vi "CalcSides.vi"(7 "Garden":u8[][](array[numeric]), 11 "Cluster":T1) -> (3 "Numeric":u64)   [LabVIEW 2023, in "2024_12.lvclass"]
uses:
  2024_12.lvclass
panel:
  out "Array":bool[][](array[boolean])
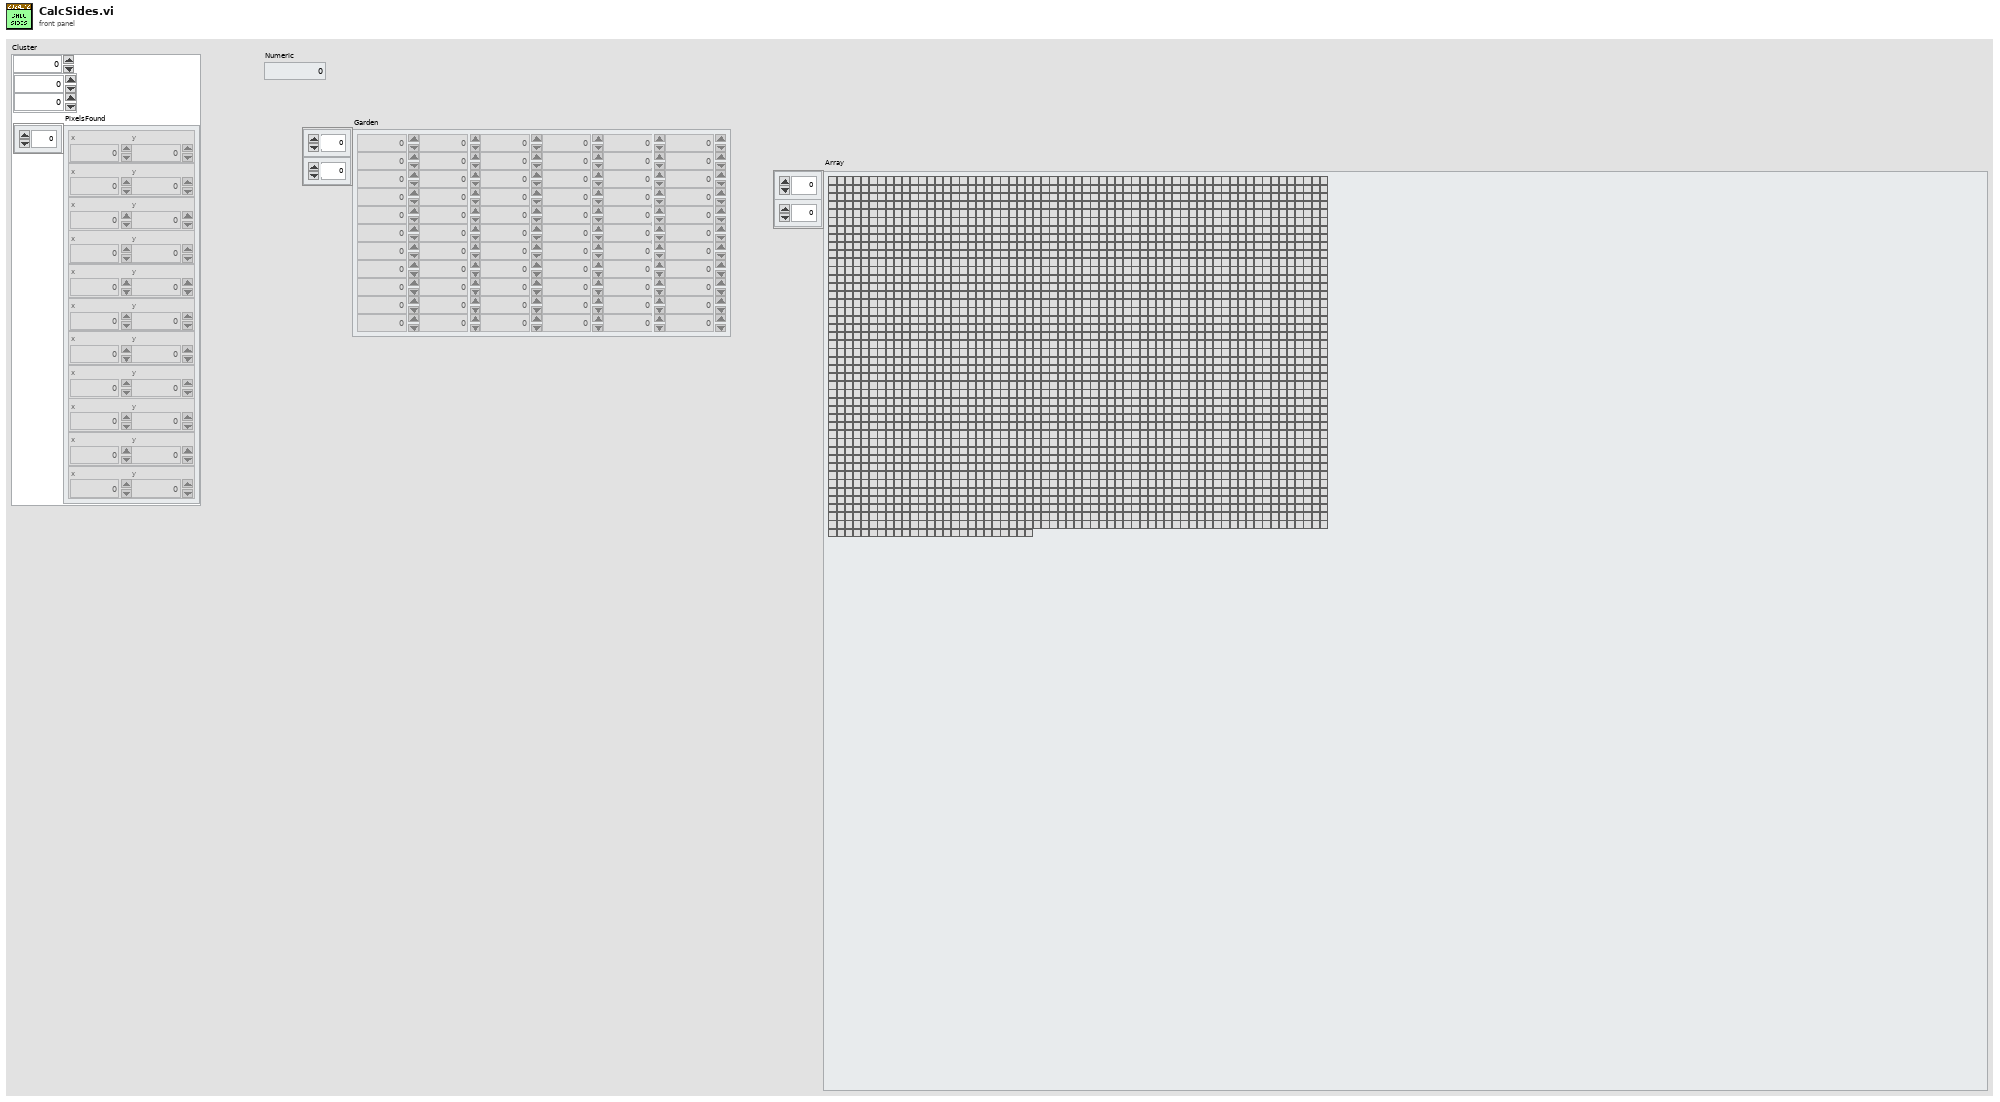
[diagram p1: front panel]
types:
  T1 = cluster{"Numeric":u8, "Cluster":cluster{"Numeric":i32, "Numeric":i32}, "PixelsFound":cluster{"x":i32, "y":i32}[]}
  T2 = cluster{"Start Position":cluster{"x":i32, "y":i32}, enum16{"Left", "Up", "Right", "Down"}, i32}
  T3 = cluster{"Start Position":cluster{"x":i32, "y":i32}, enum16{"Left", "Up", "Right", "Down"}, i32}[]
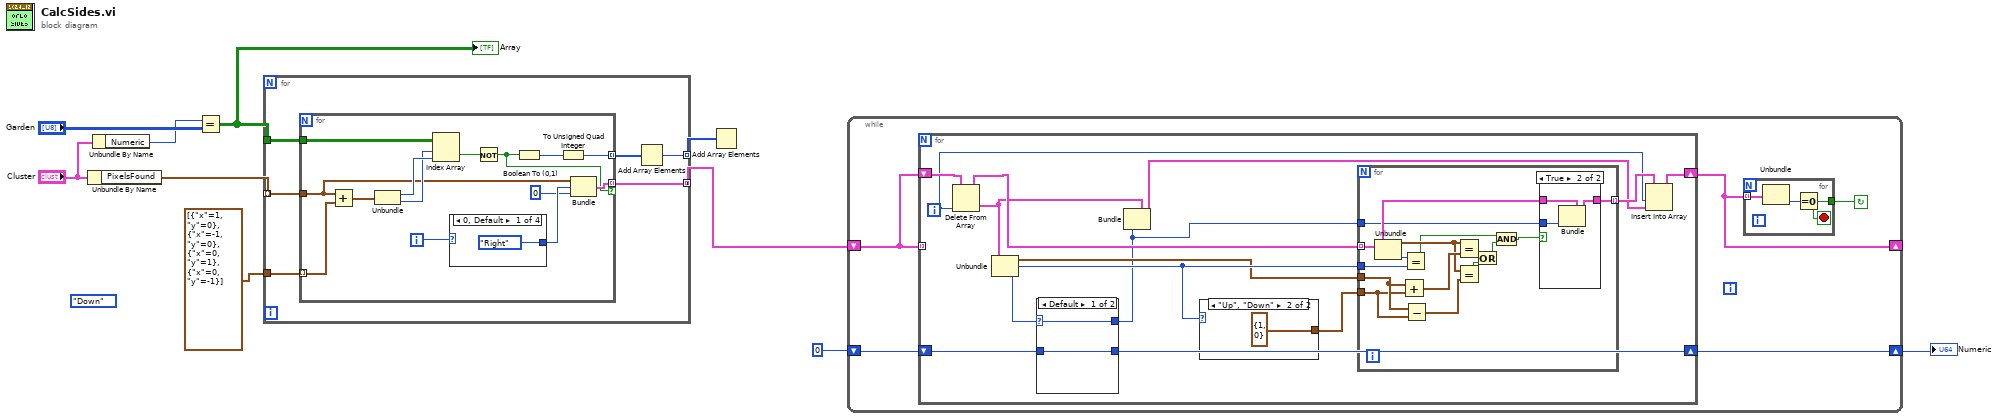
[diagram p0: block diagram]
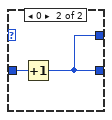
[diagram p2: hidden frame]
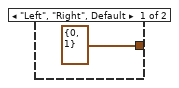
[diagram p4: hidden frame]
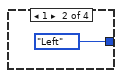
[diagram p5: hidden frame]
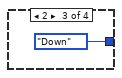
[diagram p6: hidden frame]
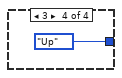
[diagram p7: hidden frame]
diagram:
  (unwired) enum16{"Left", "Up", "Right", "Down"}."Down"
  n1 = Unbundle By Name("Cluster") -> ("PixelsFound"=w10:cluster{"x":i32, "y":i32}[])
  n2 = Unbundle By Name("Cluster") -> ("Numeric"=w7:u8)
  n3 = Equal?(x=w7, y="Garden") -> (x = y?=w4:bool[][])
  "Array" <- w4
  n4 = for {
    tunnel: w10 -> [w15] mode=indexing
    tunnel: w4 -> [w16]
    tunnel: cluster{"x":i32, "y":i32}[] [{"x"=1, "y"=0}, {"x"=-1, "y"=0}, {"x"=0, "y"=1}, {"x"=0, "y"=-1}] ("PixelsFound") -> [w14]
    tunnel: [w12] -> w5 mode=indexing
    tunnel: [w11] -> w3 mode=concatenating
    n5 = for {
      tunnel: w16 -> [w30]
      tunnel: w15 -> [w21]
      tunnel: w14 -> [w29] mode=indexing
      tunnel: [w23] -> w13 mode=indexing
      tunnel: [w19] -> w11 mode=indexing if=w18
      i -> [w22]
      n6 = Add(x=w21, y=w29) -> (x+y=w28:cluster{"x":i32, "y":i32})
      n7 = Unbundle(w28) -> ("x"=w27:i32, "y"=w26:i32)
      n8 = Index Array(array=w30, index (row)=w26, index (col)=w27) -> (element=w25:bool)
      n9 = case shown="0, Default" w22 {
        tunnel: [enum16{"Left", "Up", "Right", "Down"}."Right" enum16{"Left", "Up", "Right", "Down"}."Left" enum16{"Left", "Up", "Right", "Down"}."Down" enum16{"Left", "Up", "Right", "Down"}."Up"] -> w20
        frame 0, Default {
        }
        frame 1 {
        }
        frame 2 {
        }
        frame 3 {
        }
      }
      n10 = Not(x=w25) -> (.not. x?=w18:bool)
      n11 = Boolean To (0,1)(Boolean=w18) -> (0, 1=w24:i16)
      n12 = To Unsigned Quad Integer(1:w24) -> (0:w23:u64)
      n13 = Bundle("Start Position"=w21, w20, 0) -> (w19:T2)  [unwired: 1 in]
    }
    n14 = Add Array Elements(numeric array=w13) -> (sum=w12:u64)
  }
  n15 = Add Array Elements(numeric array=w5) -> ()  [unwired: 1 out]
  n16 = while {
    shift-right: [w36] -> _
    shift-left: w3 -> [w38]
    shift-right: [w37] -> w1
    shift-left: 0 ("index") -> [w39]
    stop <- w35 continue-if-true
    n17 = for {
      tunnel: w38 -> [_] mode=indexing
      shift-right: [w48] -> w36
      shift-left: w38 -> [w50]
      shift-right: [w43] -> w37
      shift-left: w39 -> [w51]
      i -> [w47]
      n18 = Delete From Array(array=w50, index=w47) -> (deleted portion=w46:T2, array with subset deleted=w49:T3)  [unwired: 1 in]
      n19 = Unbundle(w46) -> ("Start Position"=w55:cluster{"x":i32, "y":i32}, w56:enum16{"Left", "Up", "Right", "Down"}, w52:i32)
      n20 = case shown="Default" w52 {
        selector: w52 -> [w57 _]
        tunnel: w51 -> [w58 w60]
        tunnel: [w58 w59] -> w43
        tunnel: [w57 w59] -> w44
        frame Default {
        }
        frame 0 {
          n21 = Increment(x=w60) -> (x+1=w59:i32)
        }
      }
      n22 = Bundle(cluster=w46, w44) -> (w45:T2)  [unwired: 2 in]
      n23 = case shown="\"Up\", \"Down\"" w56 {
        tunnel: [cluster{"x":i32, "y":i32} {"x"=0, "y"=1} ("Start Position") cluster{"x":i32, "y":i32} {"x"=1, "y"=0} ("Start Position")] -> w54
        frame "Left", "Right", Default {
        }
        frame "Up", "Down" {
        }
      }
      n24 = for {
        tunnel: w49 -> [w63] mode=indexing
        tunnel: w56 -> [w74]
        tunnel: w55 -> [w73]
        tunnel: w54 -> [w72]
        tunnel: [w62] -> w53 mode=indexing
        tunnel: w44 -> [w61]
        n25 = Unbundle(w63) -> ("Start Position"=w70:cluster{"x":i32, "y":i32}, w75:enum16{"Left", "Up", "Right", "Down"})  [unwired: 1 out]
        n26 = Add(x=w73, y=w72) -> (x+y=w71:cluster{"x":i32, "y":i32})
        n27 = Equal?(x=w75, y=w74) -> (x = y?=w66:bool)
        n28 = Subtract(x=w73, y=w72) -> (x-y=w69:cluster{"x":i32, "y":i32})
        n29 = Equal?(x=w70, y=w71) -> (x = y?=w68:bool)
        n30 = Equal?(x=w70, y=w69) -> (x = y?=w67:bool)
        n31 = Or(x=w68, y=w67) -> (x .or. y?=w65:bool)
        n32 = And(x=w66, y=w65) -> (x .and. y?=w64:bool)
        n33 = case shown="True" w64 {
          tunnel: w63 -> [w76 w79]
          tunnel: [w76 w78] -> w62
          tunnel: w61 -> [_ w77]
          frame False {
          }
          frame True {
            n34 = Bundle(cluster=w79, w77) -> (w78:T2)  [unwired: 2 in]
          }
        }
      }
      n35 = Insert Into Array(array=w53, index=w47, new element=w45) -> (w48:T3)
    }
    n36 = for {
      tunnel: w36 -> [w42] mode=indexing
      tunnel: [w40] -> w35
      stop <- w40 stop-if-true
      n37 = Unbundle(w42) -> (w41:i32)  [unwired: 2 out]
      n38 = Equal To 0?(x=w41) -> (x = 0?=w40:bool)
    }
  }
  "Numeric" <- w1
